vi "lv_bots_launcher.vi"() -> ()   [LabVIEW 2023]
uses:
  f91d349e-c54a-4875-81a0-e573ea4344d8.vi
panel:
  in  "LV Bots Example AI Agent":bool=TRUE
  in  "LV Bots MCP Server":bool=TRUE
  # "LV Bots Launcher"
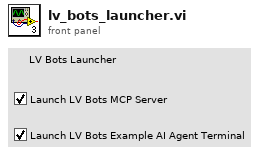
[diagram p1: front panel]
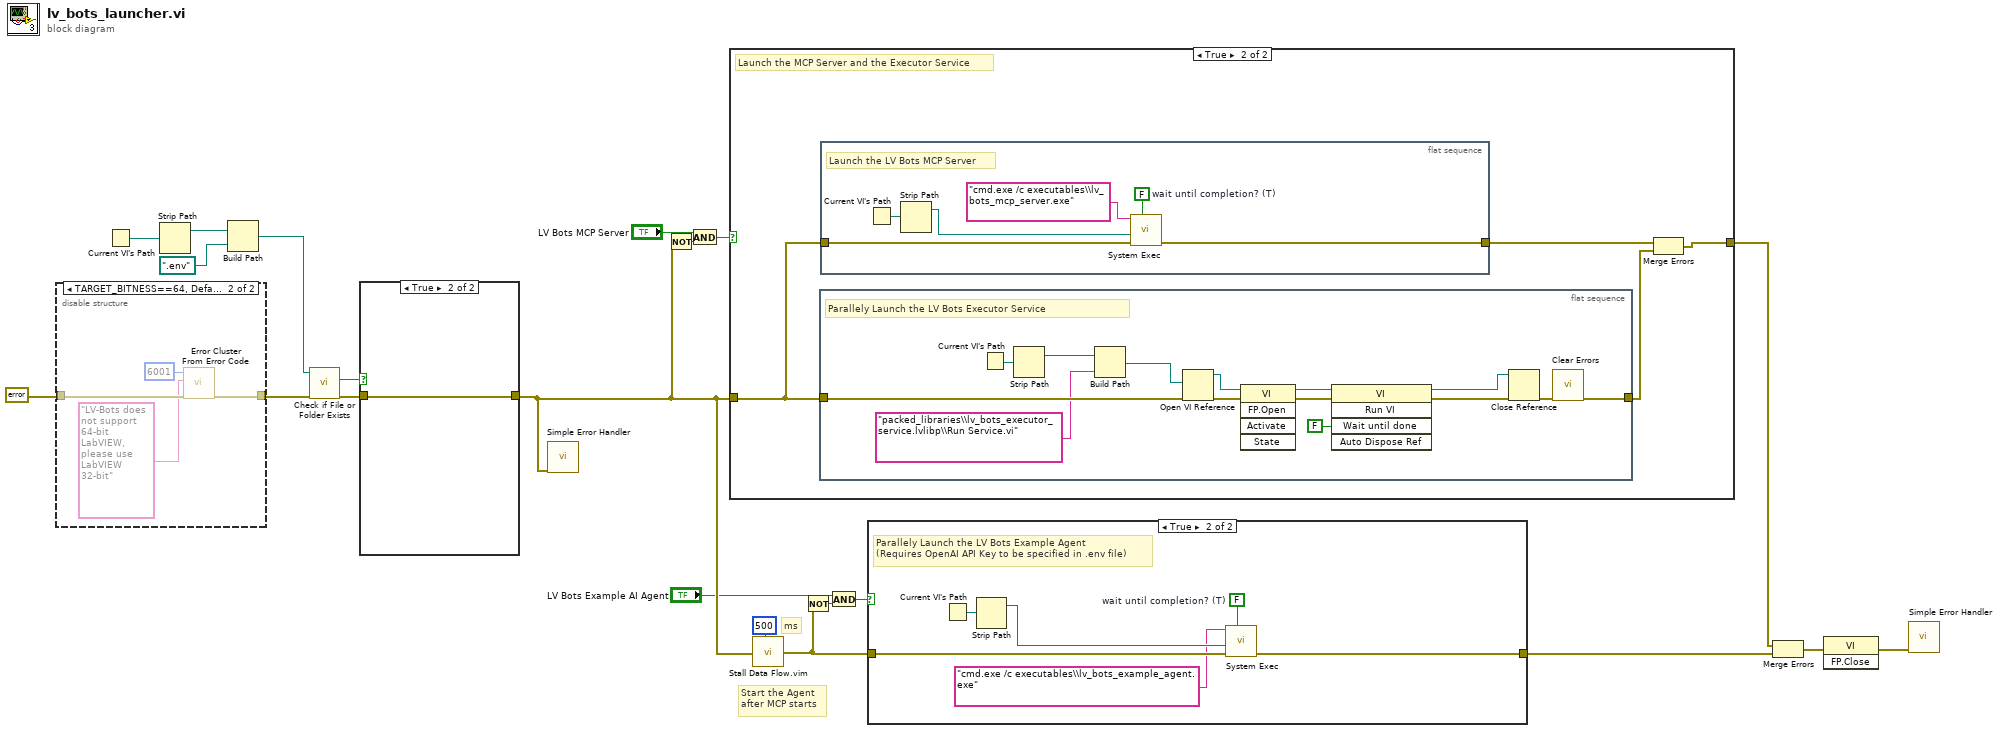
[diagram p0: block diagram]
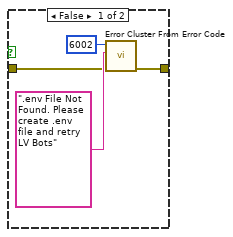
[diagram p2: hidden frame]
diagram:
  # "ms"
  # "Start the Agent\nafter MCP starts"
  n1 = disable-structure shown="TARGET_BITNESS==64, Default" {
    disable-tunnel: errorcluster {"status"=FALSE, "code"=0, "source"=""} ("error constant") -> [w22 w26]
    disable-tunnel: [w22 w23] -> w15
    frame condition #0 (active) {
    }
    frame condition #1 {
      n2 = call <vilib>:"Error Cluster From Error Code.vi"("error in (no error)"=w26, "error message (\"\")"="LV-Bots does not support 64-bit LabVIEW, please use LabVIEW 32-bit" ("error message (\"\")"), "error code (0)"=6001) -> ("error out"=w23:errorcluster)  [unwired: 6 in]
    }
  }
  n3 = Current VI's Path() -> (path=w19:path)
  n4 = Strip Path(path=w19) -> (stripped path=w18:path)  [unwired: 1 out]
  n5 = Build Path(base path=w18, name or relative path=path ".env") -> (appended path=w16:path)
  n6 = call <vilib>:"Check if File or Folder Exists.vi"("error in (no error)"=w15, "path"=w16) -> ("error out"=w14:errorcluster, "file or folder exists?"=w13:bool)  [unwired: 7 in, 1 out]
  n7 = case shown="True" w13 {
    tunnel: [w28 w31] -> w10
    tunnel: w14 -> [w27 w31]
    frame False {
      n8 = call <vilib>:"Error Cluster From Error Code.vi"("error in (no error)"=w27, "error message (\"\")"=".env File Not Found. Please create .env file and retry LV Bots" ("error message (\"\")"), "error code (0)"=6002) -> ("error out"=w28:errorcluster)  [unwired: 6 in]
    }
    frame True {
    }
  }
  n9 = call <vilib>:"Simple Error Handler.vi"("error in (no error)"=w10) -> ()  [unwired: 4 in, 5 out]
  n10 = Not(x=w10) -> (.not. x?=w6:bool)
  n11 = And(x="LV Bots MCP Server", y=w6) -> (x .and. y?=w12:bool)
  n12 = case shown="True" w12 {
    tunnel: w10 -> [w32 w36]
    tunnel: [w32 w33] -> w3
    frame False {
    }
    frame True {
      # "Launch the MCP Server and the Executor Service"
      n13 = flat-sequence {
        tunnel: w36 -> [w56]
        tunnel: [w43] -> w34
        frame #0 {
          # "Parallely Launch the LV Bots Executor Service"
          n14 = Current VI's Path() -> (path=w52:path)
          n15 = Strip Path(path=w52) -> (stripped path=w51:path)  [unwired: 1 out]
          n16 = Build Path(base path=w51, name or relative path="packed_libraries\\lv_bots_executor_service.lvlibp\\Run Service.vi" ("command line")) -> (appended path=w54:path)
          n17 = Open VI Reference(vi path=w54, error in (no error)=w56) -> (vi reference=w48:refnum<vi>, error out=w47:errorcluster)  [unwired: 4 in]
          n18 = invoke class="VI" method="FP.Open"(reference=w48, error in=w47) -> (reference out=w45:refnum<vi>, error out=w46:errorcluster)  [unwired: 3 in, 3 out]
          n19 = invoke class="VI" method="Run VI"(reference=w45, error in=w46, "Wait until done"=FALSE ("Wait Until Done")) -> (reference out=w50:refnum<vi>, error out=w49:errorcluster)  [unwired: 2 in, 3 out]
          n20 = Close Reference(reference=w50, error in (no error)=w49) -> (error out=w44:errorcluster)
          n21 = call <vilib>:"Clear Errors.vi"("error in (no error)"=w44) -> ("error out"=w43:errorcluster)  [unwired: 5 in, 1 out]
        }
      }
      n22 = flat-sequence {
        tunnel: w36 -> [w42]
        tunnel: [w37] -> w35
        frame #0 {
          w38 = FALSE  # wait until completion? (T)
          # "Launch the LV Bots MCP Server"
          n23 = Current VI's Path() -> (path=w40:path)
          n24 = Strip Path(path=w40) -> (stripped path=w39:path)  [unwired: 1 out]
          n25 = call <vilib>:"System Exec.vi"("wait until completion? (T)"=w38, "error in (no error)"=w42, "working directory"=w39, "command line"="cmd.exe /c executables\\lv_bots_mcp_server.exe") -> ("error out"=w37:errorcluster)  [unwired: 4 in, 3 out]
        }
      }
      n26 = Merge Errors(w35, w34) -> (w33:errorcluster)
    }
  }
  n27 = call "Stall Data Flow.vim"("value in"=w10, "milliseconds to wait"=u32 500) -> ("value out"=w9:errorcluster)  [unwired: 1 out]
  n28 = Not(x=w9) -> (.not. x?=w5:bool)
  n29 = And(x="LV Bots Example AI Agent", y=w5) -> (x .and. y?=w7:bool)
  n30 = case shown="True" w7 {
    tunnel: w9 -> [w57 w63]
    tunnel: [w57 w58] -> w4
    frame False {
    }
    frame True {
      w59 = FALSE  # wait until completion? (T)
      # "Parallely Launch the LV Bots Example Agent\n(Requires OpenAI API Key to be specified in .env file)"
      n31 = Current VI's Path() -> (path=w62:path)
      n32 = Strip Path(path=w62) -> (stripped path=w61:path)  [unwired: 1 out]
      n33 = call <vilib>:"System Exec.vi"("wait until completion? (T)"=w59, "error in (no error)"=w63, "working directory"=w61, "command line"="cmd.exe /c executables\\lv_bots_example_agent.exe") -> ("error out"=w58:errorcluster)  [unwired: 4 in, 3 out]
    }
  }
  n34 = Merge Errors(w3, w4) -> (w2:errorcluster)
  n35 = invoke class="VI" method="FP.Close"(error in=w2) -> (error out=w1:errorcluster)  [unwired: 2 in, 2 out]
  n36 = call <vilib>:"Simple Error Handler.vi"("error in (no error)"=w1) -> ()  [unwired: 4 in, 5 out]
